vi "[GV]_Platform Data.vi"() -> ()   [LabVIEW 2016]
panel:
  out "Platform Data":u32[](array[numeric])
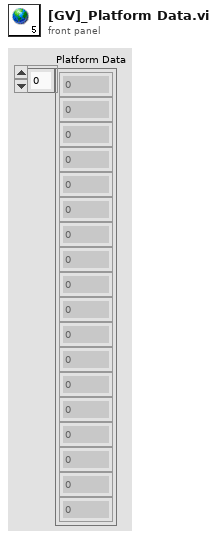
[diagram p1: front panel]
diagram:
